vi "Controller_TCrane_MoreData.vi"() -> ()   [LabVIEW 2009]
uses:
  <vilib>/Platform/TimedLoop/XDataNode/nitl_modes.ctl
  Instance           2 23Saved   OpenLoop_TCrane .vi
  <vilib>/Platform/TimedLoop/XDataNode/XDataNode.xnode
  <vilib>/Platform/TimedLoop/XDataNode/loadlvalarms.vi
  <vilib>/Platform/TimedLoop/XDataNode/timing_clust.ctl
  <vilib>/Platform/TimedLoop/XDataNode/wakeup.ctl
  Instance           3 23Saved   OpenLoop_TCrane .vi
  Instance           4 23Saved   OpenLoop_TCrane .vi
  Instance           5 23Saved   OpenLoop_TCrane .vi
  <vilib>/Utility/file.llb/Write To Spreadsheet File (DBL).vi
  <vilib>/Utility/file.llb/Write To Spreadsheet File (string).vi
  Dependences/RTdac/RTDACUSB_TCrane.dll
  <vilib>/Platform/TimedLoop/XDataNode/XDNodeRunTimeDep.lvlib
panel:
  in  "Start saving":bool
  in  "Tab Control":T1(tab)
  out "Controller Description":string
  in  "Motors on":bool caption="Motors"
  out "X displacement chart":dbl(graph)
  out "Y displacement chart":dbl(graph)
  out "Z displacement chart":dbl(graph)
  out "XY Graph":cluster{"Y":dbl[], "Y":dbl[]}[](graph)
  out "Alpha":dbl
  out "Beta":dbl
  in  "Controller:":u8(ring) items=["None", "P (Tracking)", "Self Event Triggered from ED"]
  in  "X":dbl
  in  "Stop Controller":bool
  in  "T":dbl min=0.0 max=3.14 step=0.05
  in  "Z":dbl
  in  "Referense Slide X":dbl(slide) scale=0.0..50.0
  in  "Referense Slide T":dbl(slide) scale=0.0..3.14
  in  "Referense Slide Z":dbl(slide) scale=0.0..100.0
  in  "Cont Switch X":bool
  in  "Cont Switch T":bool
  in  "Cont Switch Z":bool
  in  "stop 2":bool
  in  "Home":bool
  in  "Reset angles":bool
  in  "Motors off":bool
  in  "Saving":bool
  in  "Stop saving":bool
  out "current time":timestamp
  out "Timestamp":dbl format="%#.12g"
  out "Path":path
  out "X Scope":dynamicdata(graph)
  out "Theta Scope":dynamicdata(graph)
  out "Z Scope":dynamicdata(graph)
  out "Waveform Chart":i32(graph)
  out "Counter pulses":dbl format="%#.12g"
  out "Encoder X":dbl format="%#.12g"
  in  "X-axis control":dbl(slide) scale=-1.0..1.0
  in  "X-Motor On/Off":bool
  out "X - Motor On/Off":bool
  out "Numeric":dbl
  out "No of detected boards":dbl
  out "Logic version":dbl
  out "Last error":string
  in  "Theta-angle control":dbl(slide) scale=-1.0..1.0
  in  "T-Motor On/Off":bool
  out "Theta - Motor On/Off":bool
  out "Numeric 2":dbl
  in  "Z-axis control":dbl(slide) scale=-1.0..1.0
  in  "Z-Motor On/Off":bool
  out "Z - Motor On/Off":bool
  out "Numeric 3":dbl
  out "Encoder Theta":dbl format="%#.12g"
  out "Encoder Z":dbl format="%#.12g"
  out "Encoder Alfa":dbl format="%#.12g"
  out "Encoder Beta":dbl format="%#.12g"
  in  "Limit flags":T2(radio)=enum."Radio Selection 2"
  in  "Therm flags":T3(radio)=enum."Radio Selection 2"
  in  "Stop motors":bool
  out "X-axis therm flag":bool
  out "T-angle therm flag":bool
  out "Z-axis therm flag":bool
  out "X-axis limit flag":bool
  out "T-angle limit flag":bool
  out "Z-axis limit flag":bool
  in  "Reset encoders":bool
  out "RESET value":dbl format="%#.12g"
  in  "Soft limit flags":bool=TRUE
  in  "k 1":dbl=0.4 step=0.1
  in  "k 2":dbl=0.4 step=0.1
  in  "Mode":T4=enum."Discard missed periods, maintain original phase"
  out "Sample time [ms]":dbl format="%#.12g"
  out "Self event trigerred Enabled":bool
  out "Event interval":dbl format="%#.12g"
  out "u2":sgl
  out "u1":sgl
  out "Event indicator":bool
  out "Packet Total":u32
  out "Packet Success":u32
  out "TimestampSymb":u32
  out "X Reference":sgl
  out "Y Reference":sgl
  out "X Scope ED":dynamicdata(graph)
  out "Waveform Chart 2":dbl(graph)
  out "Theta Scope ED":dynamicdata(graph)
  out "x1":sgl(graph)
  out "x2":sgl(graph)
  out "x5":sgl(graph)
  out "x6":sgl(graph)
  out "Current Ref Z":dbl
  out "Current Ref X":dbl
  out "Current Ref T":dbl
  in  "Offset Beta":dbl
  in  "Offset Alpha":dbl
  # "RT-DAC/USB status"
  # "Tower Crane motor control"
  # "Controller Parameters"
  # "Default Controllers"
  # "Self Triggered Controller"
  # "Performance Evaluation"
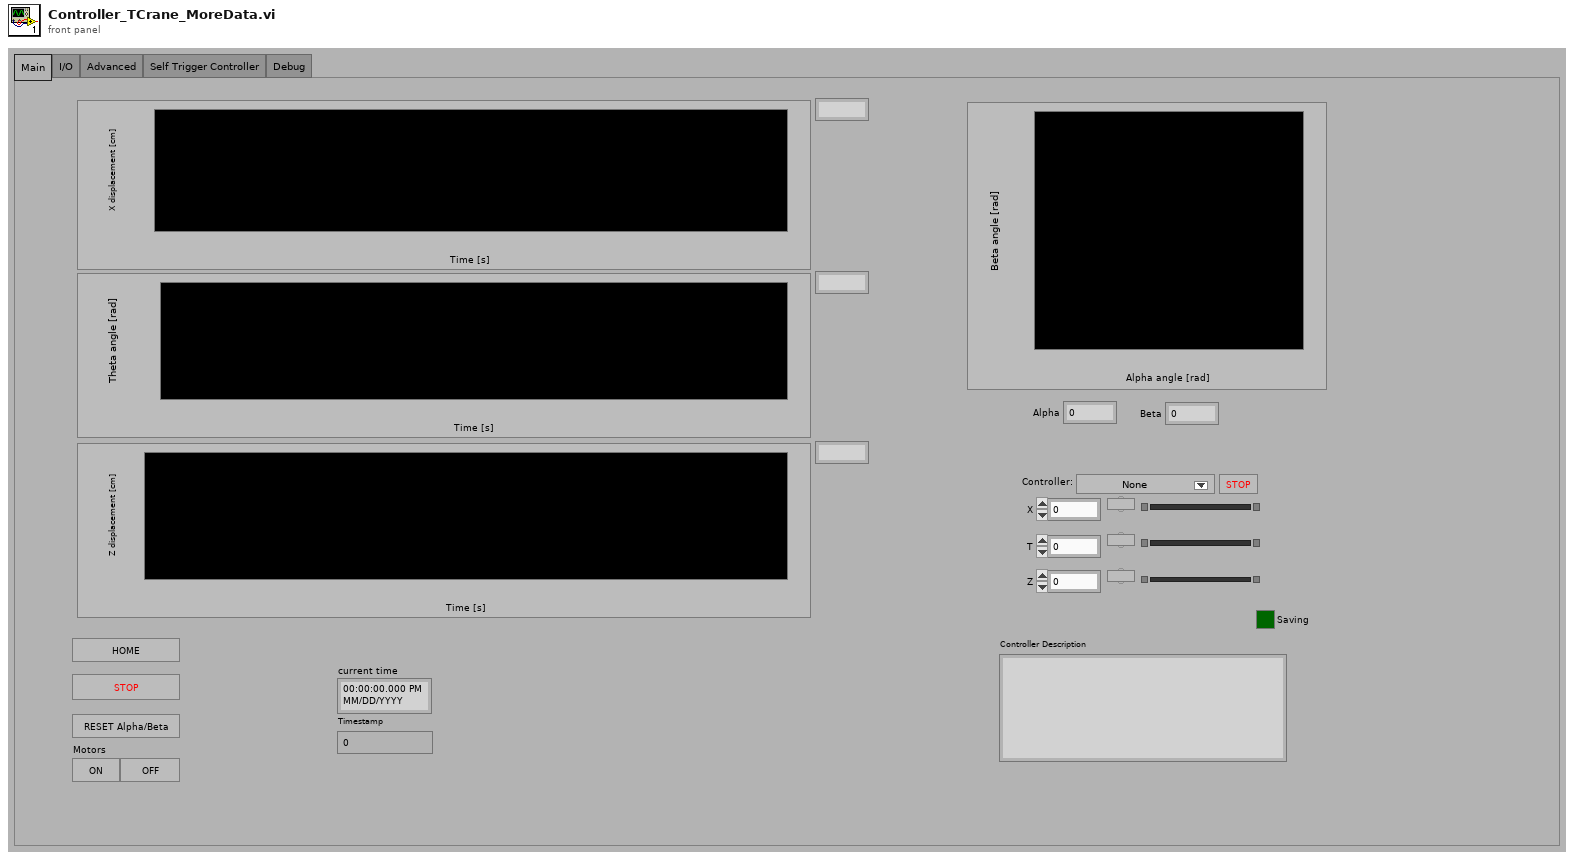
[diagram p1: front panel]
types:
  T1 = enum32{"Main", "I/O", "Advanced", "Self Trigger Controller", "Debug"}
  T2 = enum32{"Set limit flags to:", "Radio Selection 2"}
  T3 = enum32{"Set therm flags to:", "Radio Selection 2"}
  T4 = typedef "XDNodeRunTimeDep.lvlib/nitl_modes.ctl" = enum32{"No Change", "Process missed periods, maintain original phase", "Discard missed periods, maintain original phase", "Process missed periods, ignore original phase", "Discard missed periods, ignore original phase"}
  T5 = typedef "XDNodeRunTimeDep.lvlib/timing_clust.ctl" = cluster{"Expected End [f-1]":u64, "Actual End [f-1]":u64, "Finished Late? [f-1]":bool, "Expected End [i-1]":u64, "Actual End [i-1]":u64, "Finished Late? [i-1]":bool, "Expected Start [i]":u64, "Actual Start [i]":u64, "Expected Start [f]":u64, "Actual Start [f]":u64, "Source Name":string, "Structure Name":string, "Period":i64, "Deadline":i64, "Offset":i64, "Start":i64, "Priority":i32, "Timeout":i32, "Mode":T4, "Wakeup Reason":T6, "Error":errorcluster, "Source Type":string, "Secondary Source Type":string, "Global End Time":u64, "Global Start Time":u64, "Frame Duration":u64, "Iteration Duration":u64, "Assigned CPU":i32, "I/O Scan Engine Mode":u32}
  T6 = typedef "XDNodeRunTimeDep.lvlib/wakeup.ctl" = enum32{"Normal", "Aborted", "Asynchronous wakeup", "Timing source error", "Timed loop error", "Timeout"}
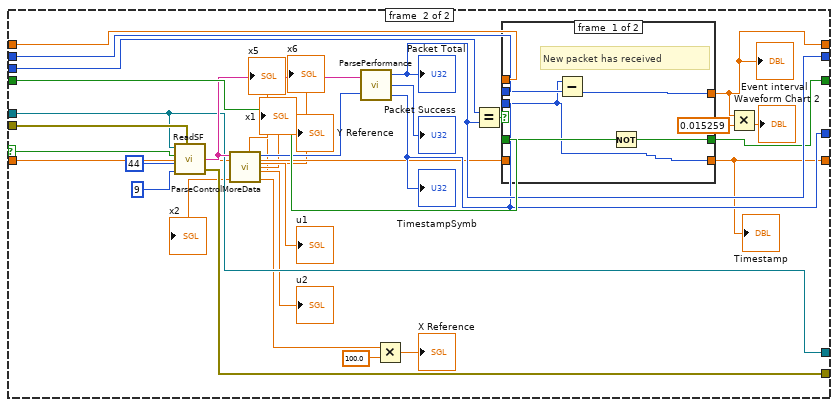
[diagram p2: hidden frame]
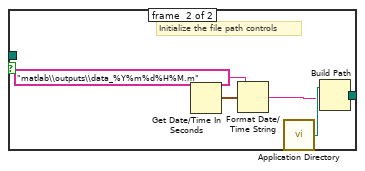
[diagram p4: hidden frame]
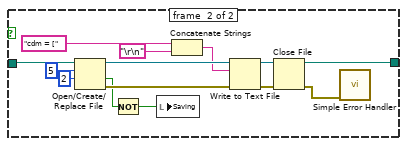
[diagram p5: hidden frame]
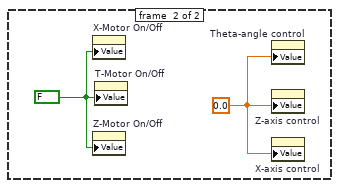
[diagram p6: hidden frame]
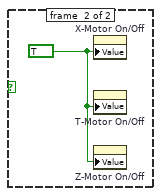
[diagram p7: hidden frame]
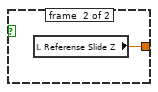
[diagram p8: hidden frame]
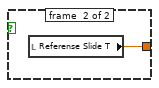
[diagram p9: hidden frame]
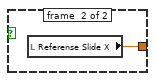
[diagram p10: hidden frame]
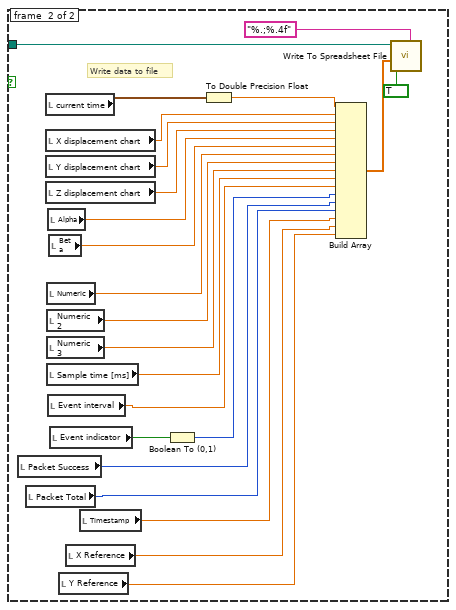
[diagram p11: hidden frame]
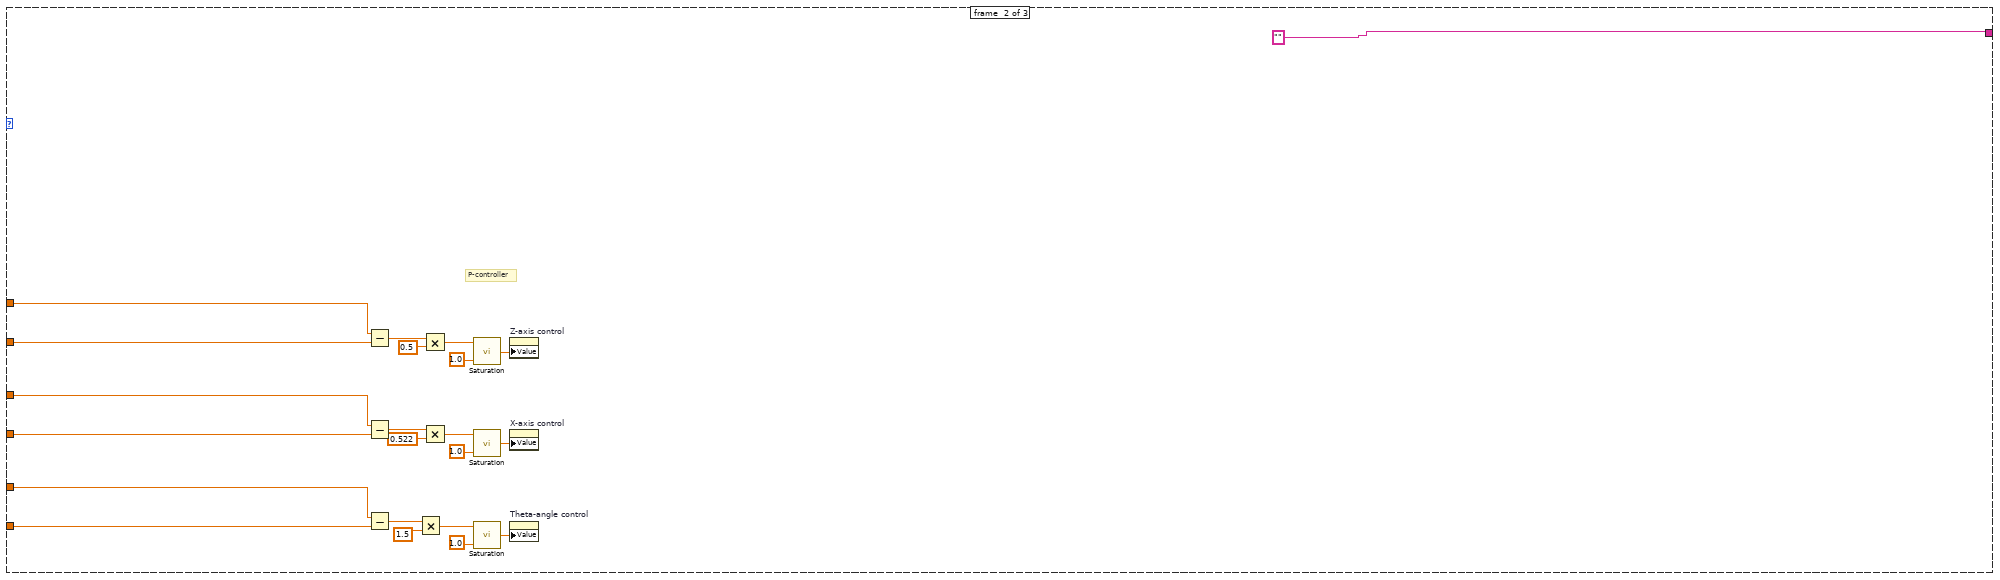
[diagram p12: hidden frame]
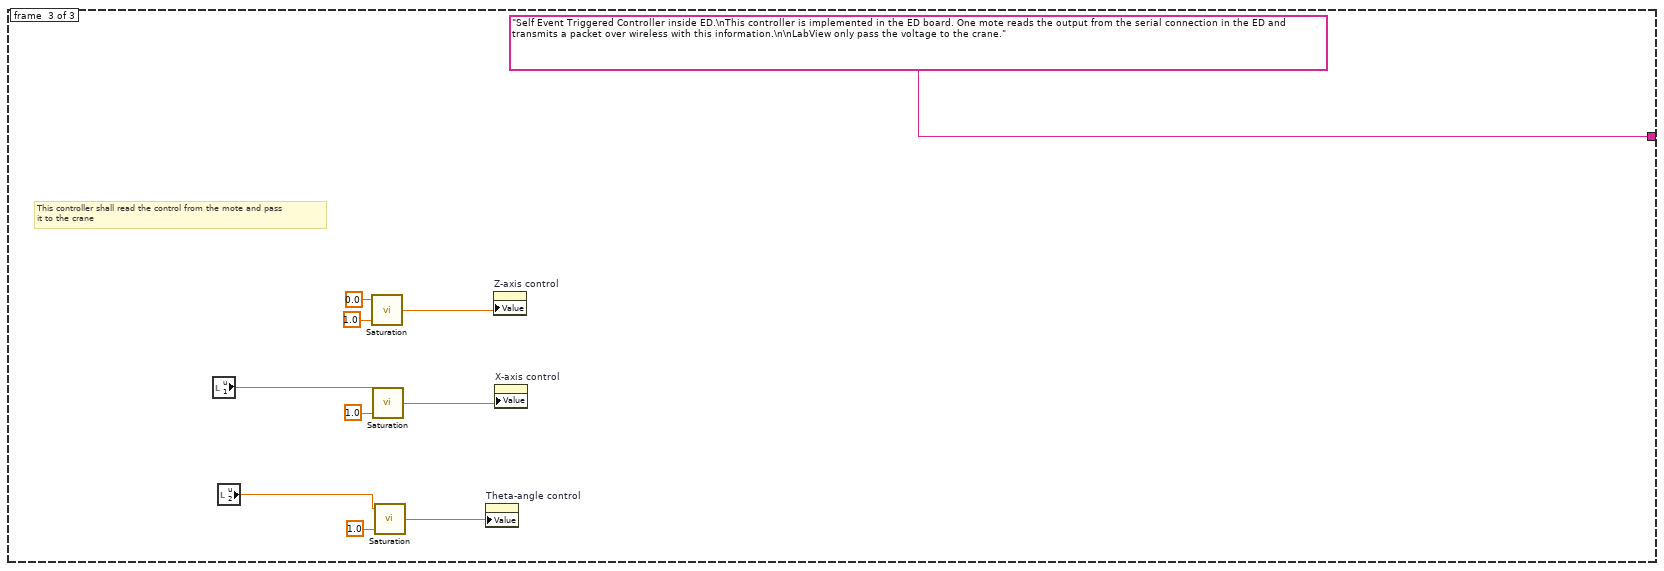
[diagram p13: hidden frame]
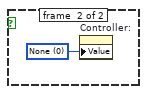
[diagram p14: hidden frame]
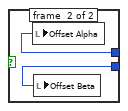
[diagram p15: hidden frame]
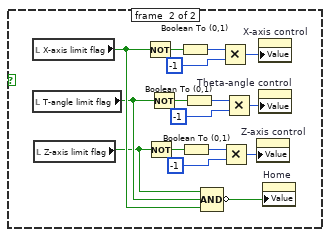
[diagram p16: hidden frame]
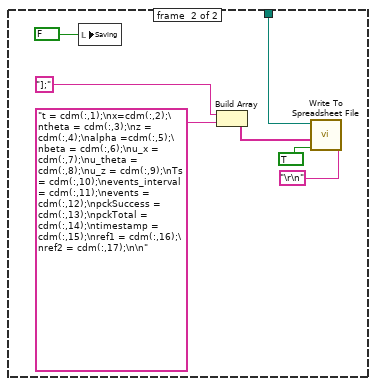
[diagram p17: hidden frame]
diagram:
  (unwired) 0.0
  (unwired) 0.0
  w10 = 0.0
  # "Initialize the file path controls"
  # "Initialize the file path controls"
  n1 = Get Date/Time In Seconds() -> (seconds since 1Jan1904=w9:timestamp)
  n2 = dll-call lib="C:/Documents and Settings/student/Desktop/crane controller/Dependences/RTdac/RTDACUSB_TCrane.dll" fn="RTDACUSB_NoOfDetectedBoards" ("PlxApi.dll:PlxBusIopWrite")() -> ("pNoOfDetectedBoards"=w23:i32)  [unwired: 5 in, 2 out]
  "No of detected boards" <- w23
  n3 = Format Date/Time String(time format string (%c)="matlab\\outputs\\data_%Y%m%d%H%M.m", seconds (now)=w9) -> (date/time string=w6:string)  [unwired: 1 in]
  n4 = call <vilib>:"Application Directory.vi"() -> ("Application Directory"=w17:path)
  n5 = Build Path(base path=w17, name or relative path=w6) -> (appended path=w7:path)
  n6 = Less?(x=w23, y=1) -> (x < y?=w22:bool)
  n7 = local write "Path"(w7) -> ()
  n8 = call "Display Message to User"("Enable"=w22) -> ("OK"=w11:bool)  [unwired: 9 in, 1 out]
  n9 = Get Date/Time In Seconds() -> (seconds since 1Jan1904=w4:timestamp)
  n10 = call "OpenSF.vi"() -> ("error out"=w15:errorcluster, "connection ID"=w16:refnum<k5>)  [unwired: 1 out]
  n11 = Format Date/Time String(time format string (%c)="matlab\\outputs\\data_%Y%m%d%H%M.m", seconds (now)=w4) -> (date/time string=w2:string)  [unwired: 1 in]
  n12 = call <vilib>:"Application Directory.vi"() -> ("Application Directory"=w5:path)
  n13 = while {
    tunnel: w16 -> [w51]
    tunnel: w15 -> [w50]
    tunnel: [w49] -> w14
    tunnel: [w48] -> w13
    shift-right: [w40] -> _
    shift-left: FALSE -> [w45]
    shift-right: [w44] -> _
    shift-left: _ -> [w43]
    shift-right: [w42] -> _
    shift-left: _ -> [w41]
    shift-right: [w38] -> _
    shift-left: w10 -> [w39]
    shift-right: [w25] -> _
    shift-left: w10 -> [w24]
    stop <- TRUE continue-if-true
    # "Feed control signals, reference signals and measurements into the scopes"
    # "Read data from the Serial Forwarer (motes)"
    n14 = local read "Self event trigerred Enabled"() -> (w47:bool)
    n15 = case shown="True" w47 {
      selector: w47 -> [_ w65]
      tunnel: w51 -> [w57 w83]
      tunnel: w50 -> [w56 w88]
      tunnel: [w57 w83] -> w49
      tunnel: [w56 w89] -> w48
      tunnel: w45 -> [w55 w86]
      tunnel: [w55 w76] -> w40
      tunnel: [w54 w74] -> w44
      tunnel: w43 -> [w54 w73]
      tunnel: [_ w79] -> w42
      tunnel: w41 -> [_ w78]
      tunnel: [w53 w59] -> w38
      tunnel: w39 -> [w53 w75]
      tunnel: [w52 w67] -> w25
      tunnel: w24 -> [w52 w66]
      frame #0 {
      }
      frame #1 {
        n16 = call "ReadSF.vi"("connection ID in"=w83, "enabled"=w65, "bytes to read"=44 ("f"), "header size"=9 ("bytes to read"), "error in"=w88) -> ("string"=w85:string, "error out"=w89:errorcluster)  [unwired: 1 out]
        n17 = call "ParseControlMoreData.vi"("data out"=w85) -> ("ref1"=w69:sgl, "u2"=→"u2":sgl, "u1"=→"u1":sgl, "Bytes read"=w72:i32, "ref2"=→"Y Reference":sgl, "x1"=→"x1":sgl, "x2"=→"x2":sgl, "x5"=→"x5":sgl, "x6"=→"x6":sgl)
        n18 = call "ParsePerformance.vi"("data out"=w85, "offset"=w72) -> ("pckTotal"=w79:u32, "pckSuccess"=→"Packet Success":u32, "timestamp"=w74:u32)
        "Packet Total" <- w79
        "TimestampSymb" <- w74
        n19 = Multiply(x=w69, y=sgl 100.0) -> (x*y=→"X Reference":sgl)
        n20 = Equal?(x=w78, y=w79) -> (x = y?=w77:bool)
        n21 = case shown="True" w77 {
          tunnel: w86 -> [w94 w97]
          tunnel: [w93 w97] -> w76
          tunnel: w75 -> [_ w96]
          tunnel: [w91 w96] -> w59
          tunnel: w74 -> [w90 _]
          tunnel: w73 -> [w92 _]
          tunnel: [w90 w95] -> w67
          tunnel: w66 -> [_ w95]
          frame #0 {
            # "New packet has received"
            n22 = Subtract(x=w90, y=w92) -> (x-y=w91:u32)
            n23 = Not(x=w94) -> (.not. x?=w93:bool)
          }
          frame #1 {
          }
        }
        "Event interval" <- w59
        "Timestamp" <- w67
        n24 = Multiply(x=w59, y=0.015259) -> (x*y=→"Waveform Chart 2":dbl)
      }
    }
    "Event indicator" <- w40
    n25 = local read "X Reference"() -> (w33:sgl)
    n26 = local read "Y Reference"() -> (w27:sgl)
    n27 = local read "Y displacement chart"() -> (w30:dbl)
    n28 = local read "X displacement chart"() -> (w26:dbl)
    n29 = local read "u2"() -> (w28:sgl)
    n30 = local read "u1"() -> (w36:sgl)
    n31 = Multiply(x=w28, y=5) -> (x*y=w31:sgl)
    n32 = Multiply(x=w36, y=40) -> (x*y=w34:sgl)
    n33 = Merge Signals(w30, w27, w31) -> (→"Theta Scope ED":dynamicdata)
    n34 = Merge Signals(w26, w33, w34) -> (→"X Scope ED":dynamicdata)
  }
  n35 = Build Path(base path=w5, name or relative path=w2) -> (appended path=w1:path)
  n36 = node-c288("Mode") -> (w20:T5)  [unwired: 9 in]
  n37 = timed-loop {
    tunnel: w11 -> [w289]
    timing: w20 -> [_]
    timing-out: [_] -> w19
    shift-right: [w101] -> _
    shift-left: w1 -> [w99]
    stop <- w290 stop-if-true
    w135 = 0.00153
    w238 = 0.00153
    w276 = 1
    w136 = 0
    # "It enabled to read from the mote"
    # "Plot the values from the Wireless sensor"
    # "Stop saving of data"
    # "Turn off all the motors"
    # "Turn on all the motors"
    # "Get reference signals"
    # "Take crane to home position"
    # "Stop the controller"
    # "Feed control signals, reference signals and measurements into the scopes"
    n38 = node-c288() -> ()  [unwired: 1 in, 1 out]
    n39 = Get Date/Time In Seconds() -> (seconds since 1Jan1904=w120:timestamp)
    "current time" <- w120
    n40 = local read "Stop Controller"() -> (w141:bool)
    n41 = local read "Stop motors"() -> (w140:bool)
    n42 = Compound Arithmetic op=OR(w141, "Motors off", w140) -> (w143:bool)
    n43 = dll-call lib="C:/Documents and Settings/student/Desktop/crane controller/Dependences/RTdac/RTDACUSB_TCrane.dll" fn="RTDACUSB_Receive" ("PlxApi.dll:PlxBusIopWrite")("pLogicVersion"=w136, "pApplicationName"="TestInTeCo", "pCN1Direction"=w136, "pCN1Input"=w136, "pPWMDivider"=w136, "pPWMWidth0"=w136, "pPWMWidth1"=w136, "pPWMWidth2"=w136, "pPWMDir0"=w136, "pPWMDir1"=w136, "pPWMDir2"=w136, "pPWMBrake0"=w136, "pPWMBrake1"=w136, "pPWMBrake2"=w136, "pPWMTherm0"=w136, "pPWMTherm1"=w136, "pPWMTherm2"=w136, "pPWMThermFlag0"=w136, "pPWMThermFlag1"=w136, "pPWMThermFlag2"=w136, "pNOFlag"=w136, "pLimitActive0"=w136, "pLimitActive1"=w136, "pLimitActive2"=w136, "pLimitFlag0"=w136, "pLimitFlag1"=w136, "pLimitFlag2"=w136, "pLimit0"=w136, "pLimit1"=w136, "pLimit2"=w136, "pEncoderReset0"=w136, "pEncoderReset1"=w136, "pEncoderReset2"=w136, "pEncoderReset3"=w136, "pEncoderReset4"=w136, "pEncoderAutoResetFlag0"=w136, "pEncoderAutoResetFlag1"=w136, "pEncoderAutoResetFlag2"=w136, "pEncoder0"=w136, "pEncoder1"=w136, "pEncoder2"=w136, "pEncoder3"=w136, "pEncoder4"=w136, "pTmrCnt0_Reset"=w136, "pTmrCnt0_Mode"=w136, "pTmrCnt0_Counter"=w136) -> ("pLogicVersion"=→"Logic version":u32, "pPWMThermFlag0"=w257:u32, "pPWMThermFlag1"=w258:u32, "pPWMThermFlag2"=w259:u32, "pLimitActive0"=w237:u32, "pLimitActive1"=w235:u32, "pLimitActive2"=w236:u32, "pEncoder0"=w129:i32, "pEncoder1"=w127:i32, "pEncoder2"=w125:i32, "pEncoder3"=w204:i32, "pEncoder4"=w203:i32, "pTmrCnt0_Counter"=w281:u32)  [unwired: 37 in, 2 out]
    "Counter pulses" <- w281
    "Encoder X" <- w129
    "Encoder Theta" <- w127
    "Encoder Z" <- w125
    n44 = case shown="True" "Reset angles" {
      tunnel: w204 -> [_ w389]
      tunnel: w203 -> [_ w388]
      frame #0 {
      }
      frame #1 {
        n45 = local write "Offset Alpha"(w389) -> ()
        n46 = local write "Offset Beta"(w388) -> ()
      }
    }
    n47 = case shown="True" w143 {
      frame #0 {
      }
      frame #1 {
        w318 = 0.0 ("Theta-angle control")
        w319 = FALSE ("T-Motor On/Off")
        n48 = property on="X-Motor On/Off" class="Bool (strict)"("Value"=w319) -> ()  [unwired: 2 in, 2 out]
        n49 = property on="Z-Motor On/Off" class="Bool (strict)"("Value"=w319) -> ()  [unwired: 2 in, 2 out]
        n50 = property on="T-Motor On/Off" class="Bool (strict)"("Value"=w319) -> ()  [unwired: 2 in, 2 out]
        n51 = property on="Theta-angle control" class="Slide (strict)"("Value"=w318) -> ()  [unwired: 2 in, 2 out]
        n52 = property on="Z-axis control" class="Slide (strict)"("Value"=w318) -> ()  [unwired: 2 in, 2 out]
        n53 = property on="X-axis control" class="Slide (strict)"("Value"=w318) -> ()  [unwired: 2 in, 2 out]
      }
    }
    n54 = case shown="True" "Motors on" {
      frame #0 {
      }
      frame #1 {
        w320 = TRUE ("X-Motor On/Off")
        n55 = property on="X-Motor On/Off" class="Bool (strict)"("Value"=w320) -> ()  [unwired: 2 in, 2 out]
        n56 = property on="T-Motor On/Off" class="Bool (strict)"("Value"=w320) -> ()  [unwired: 2 in, 2 out]
        n57 = property on="Z-Motor On/Off" class="Bool (strict)"("Value"=w320) -> ()  [unwired: 2 in, 2 out]
      }
    }
    n58 = case shown="True" "Stop Controller" {
      frame #0 {
      }
      frame #1 {
        w387 = u16 0 items=["None", "P"] ("Controller:")
        n59 = property on="Controller:" class="Ring (strict)"("Value"=w387) -> ()  [unwired: 2 in, 2 out]
      }
    }
    n60 = Greater?(x=w257, y=1) -> (0:→"X-axis therm flag":bool)
    n61 = Less?(x=w237, y=1) -> (x < y?=→"X-axis limit flag":bool)
    n62 = Less?(x=w235, y=1) -> (x < y?=→"T-angle limit flag":bool)
    n63 = Less?(x=w236, y=1) -> (x < y?=→"Z-axis limit flag":bool)
    n64 = Greater?(x=w258, y=1) -> (0:→"T-angle therm flag":bool)
    n65 = Greater?(x=w259, y=1) -> (0:→"Z-axis therm flag":bool)
    n66 = Multiply(x=w125, y=0.00995) -> (x*y=→"Z displacement chart":dbl)
    n67 = Multiply(x=w127, y=0.00157) -> (x*y=→"Y displacement chart":dbl)
    n68 = Subtract(x=w204, y="Offset Alpha") -> (x-y=w132:dbl)
    "Encoder Alfa" <- w132
    n69 = Subtract(x=w203, y="Offset Beta") -> (x-y=w134:dbl)
    "Encoder Beta" <- w134
    n70 = Multiply(x=w129, y=0.00582) -> (x*y=→"X displacement chart":dbl)
    n71 = local read "Encoder Beta"() -> (w239:dbl)
    n72 = local read "Encoder Alfa"() -> (w240:dbl)
    n73 = Multiply(x=w240, y=w238) -> (x*y=w242:dbl)
    n74 = Multiply(x=w239, y=w238) -> (x*y=w241:dbl)
    n75 = To Double Precision Float(number=w281) -> (double precision float=w288:dbl)
    n76 = To Double Precision Float(number=w120) -> (double precision float=w123:dbl)
    n77 = Multiply(x=w134, y=w135) -> (x*y=→"Beta":dbl)
    n78 = while {
      shift-right: [w317] -> w122
      shift-left: _ -> [w316]
      tunnel: w123 -> [w317]
      tunnel: [w316] -> w121
      tunnel: FALSE -> [w315]
      stop <- w315 continue-if-true
    }
    n79 = Multiply(x=w132, y=w135) -> (x*y=→"Alpha":dbl)
    n80 = for {
      N: 10 -> [_]
      tunnel: w241 -> [w413]
      tunnel: w242 -> [w414]
      tunnel: [w414] -> w249 mode=indexing
      tunnel: [w413] -> w248 mode=indexing
    }
    n81 = while {
      shift-right: [w417] -> w287
      shift-left: _ -> [w416]
      tunnel: w288 -> [w417]
      tunnel: [w416] -> w286
      tunnel: FALSE -> [w415]
      stop <- w415 continue-if-true
    }
    n82 = Subtract(x=w122, y=w121) -> (x-y=w118:dbl)
    n83 = call "Convert to Dynamic Data"("Array"=w249) -> ("Dynamic Data Type"=w250:dynamicdata)  [unwired: 3 in]
    n84 = call "Convert to Dynamic Data2"("Array"=w248) -> ("Dynamic Data Type"=w252:dynamicdata)  [unwired: 3 in]
    n85 = Multiply(x=w118, y=1000.0) -> (x*y=w116:dbl)
    "Sample time [ms]" <- w116
    n86 = Subtract(x=w287, y=w286) -> (x-y=w285:dbl)
    n87 = call "Build XY Graph"("Y Input"=w252, "X Input"=w250) -> ("XY Graph"=→"XY Graph":cluster{"Y":dbl[], "Y":dbl[]}[])  [unwired: 8 in, 1 out]
    n88 = Divide(x=w285, y=40000) -> ()  [unwired: 1 out]
    n89 = Or(x=w289, y="stop 2") -> (x .or. y?=w290:bool)
    n90 = To Long Integer(number=w116) -> (32bit integer=→"Waveform Chart":i32)
    n91 = Stop(stop? (T)=w290) -> ()
    n92 = Or(x="Stop saving", y=w290) -> (x .or. y?=w213:bool)
    n93 = And(x="Saving", y=w213) -> (x .and. y?=w124:bool)
    n94 = local read "Saving"() -> (w114:bool)
    n95 = Not(x=w114) -> (.not. x?=w115:bool)
    n96 = And(x="Start saving", y=w115) -> (x .and. y?=w98:bool)
    n97 = case shown="True" w98 {
      tunnel: [w291 w292] -> w100
      tunnel: w99 -> [w291 _]
      frame #0 {
      }
      frame #1 {
        # "Initialize the file path controls"
        n98 = Get Date/Time In Seconds() -> (seconds since 1Jan1904=w295:timestamp)
        n99 = Format Date/Time String(time format string (%c)="matlab\\outputs\\data_%Y%m%d%H%M.m", seconds (now)=w295) -> (date/time string=w293:string)  [unwired: 1 in]
        n100 = call <vilib>:"Application Directory.vi"() -> ("Application Directory"=w296:path)
        n101 = Build Path(base path=w296, name or relative path=w293) -> (appended path=w292:path)
      }
    }
    "Path" <- w100
    n102 = flat-sequence {
      tunnel: [w299] -> w101
      tunnel: w98 -> [w298]
      tunnel: w100 -> [w297]
      frame #0 {
        # "Initialize saving of data"
        n103 = case shown="True" w298 {
          tunnel: w297 -> [w300 w306]
          tunnel: [w300 w303] -> w299
          frame #0 {
          }
          frame #1 {
            n104 = Open/Create/Replace File(file path (use dialog)=w306, operation (0:open)=5, access (0:read/write)=2) -> (refnum out=w312:refnum<file>, cancelled=w305:bool, error out=w309:errorcluster)  [unwired: 3 in]
            n105 = Not(x=w305) -> (.not. x?=w301:bool)
            n106 = local write "Saving"(w301) -> ()
            n107 = Concatenate Strings("cdm = [", "\r\n") -> (w308:string)
            n108 = Write to Text File(file (use dialog)=w312, text=w308, error in=w309) -> (refnum out=w311:refnum<file>, error out=w310:errorcluster)  [unwired: 1 in, 1 out]
            n109 = Close File(refnum=w311, error in=w310) -> (path=w303:path, error out=w302:errorcluster)
            n110 = call <vilib>:"Simple Error Handler.vi"("error in (no error)"=w302) -> ()  [unwired: 4 in, 5 out]
          }
        }
      }
    }
    n111 = local read "Stop Controller"() -> (w196:bool)
    n112 = local read "Stop motors"() -> (w198:bool)
    n113 = local read "T-angle limit flag"() -> (w230:bool)
    n114 = case shown="True" w124 {
      tunnel: w101 -> [_ w410]
      frame #0 {
      }
      frame #1 {
        n115 = local write "Saving"(FALSE) -> ()
        n116 = Build Array("];", "t = cdm(:,1);\nx=cdm(:,2);\ntheta = cdm(:,3);\nz = cdm(:,4);\nalpha =cdm(:,5);\nbeta = cdm(:,6);\nu_x = cdm(:,7);\nu_theta = cdm(:,8);\nu_z = cdm(:,9);\nTs = cdm(:,10);\nevents_interval = cdm(:,11);\nevents = cdm(:,12);\npckSuccess = cdm(:,13);\npckTotal = cdm(:,14);\ntimestamp = cdm(:,15);\nref1 = cdm(:,16);\nref2 = cdm(:,17);\n\n") -> (w409:string[])
        n117 = call-poly <vilib>:"Write To Spreadsheet File.vi"("delimiter (\\t)"="\r\n", "append to file? (new file:F)"=TRUE, "1D data"=w409, "file path (dialog if empty)"=w410) -> ()  [unwired: 4 in, 1 out]
      }
    }
    n118 = local read "Limit flags"() -> (w233:T2)
    n119 = local read "Soft limit flags"() -> (w209:bool)
    n120 = Or(x=w196, y=w198) -> (x .or. y?=w197:bool)
    n121 = feedback #1() -> (w155:dbl)  [unwired: 1 in]
    n122 = call "LimitFlagActionSoftLinearizedT.vi"("Soft"=w209, "Axis limit flag"=w230, "Old Control"=w155, "Global limit flag active"=w233, "Stop motors global"=w197, "Stop motor local"="T-Motor On/Off", "Axis control signal"="Theta-angle control") -> ("Slider control"=w154:dbl, "PWM Brake"=w229:u32, "PWM Direction"=w228:u32, "PWM width"=w227:u32)
    n123 = local read "Stop Controller"() -> (w193:bool)
    n124 = local read "X-axis limit flag"() -> (w220:bool)
    n125 = local read "Stop motors"() -> (w195:bool)
    n126 = local read "Soft limit flags"() -> (w208:bool)
    n127 = local read "Limit flags"() -> (w221:T2)
    n128 = local read "Stop Controller"() -> (w199:bool)
    n129 = Or(x=w193, y=w195) -> (x .or. y?=w194:bool)
    n130 = local read "Z-axis limit flag"() -> (w158:bool)
    n131 = local read "Limit flags"() -> (w224:T2)
    n132 = feedback #2() -> (w153:dbl)  [unwired: 1 in]
    n133 = call "LimitFlagActionSoftLinearizedX.vi"("Soft"=w208, "Axis limit flag"=w220, "Old Control"=w153, "Global limit flag active"=w221, "Stop motors global"=w194, "Stop motor local"="X-Motor On/Off", "Axis control signal"="X-axis control") -> ("Slider control"=w152:dbl, "PWM Brake"=w217:u32, "PWM Direction"=w216:u32, "PWM width"=w215:u32)
    n134 = local read "Cont Switch T"() -> (w162:bool)
    n135 = local read "Cont Switch X"() -> (w164:bool)
    n136 = local read "Cont Switch Z"() -> (w160:bool)
    n137 = Or(x=w199, y="Stop motors") -> (x .or. y?=w200:bool)
    n138 = case shown="False" w162 {
      tunnel: [w325 w326] -> w161
      frame #0 {
        n139 = local read "T"() -> (w325:dbl)
      }
      frame #1 {
        n140 = local read "Referense Slide T"() -> (w326:dbl)
      }
    }
    n141 = case shown="False" w164 {
      tunnel: [w327 w328] -> w163
      frame #0 {
        n142 = local read "X"() -> (w327:dbl)
      }
      frame #1 {
        n143 = local read "Referense Slide X"() -> (w328:dbl)
      }
    }
    n144 = case shown="False" w160 {
      tunnel: [w323 w324] -> w159
      frame #0 {
        n145 = local read "Z"() -> (w323:dbl)
      }
      frame #1 {
        n146 = local read "Referense Slide Z"() -> (w324:dbl)
      }
    }
    n147 = feedback #3() -> (w157:dbl)  [unwired: 1 in]
    n148 = call "LimitFlagActionSoftLinearizedZ.vi"("Soft"="Soft limit flags", "Axis limit flag"=w158, "Old Control"=w157, "Global limit flag active"=w224, "Stop motors global"=w200, "Stop motor local"="Z-Motor On/Off", "Axis control signal"="Z-axis control") -> ("Slider control"=w156:dbl, "PWM Brake"=w151:u32, "PWM Direction"=w226:u32, "PWM width"=w225:u32)
    n149 = dll-call lib="C:/Documents and Settings/student/Desktop/crane controller/Dependences/RTdac/RTDACUSB_TCrane.dll" fn="RTDACUSB_LastError" ("PlxApi.dll:PlxBusIopWrite")() -> ("dsrp"=→"Last error":string)  [unwired: 3 in, 2 out]
    n150 = Boolean To (0,1)(Boolean="Reset encoders") -> (0, 1=w246:i16)
    "RESET value" <- w246
    n151 = local read "X displacement chart"() -> (w179:dbl)
    n152 = local read "X-axis control"() -> (w173:dbl)
    n153 = local read "Y displacement chart"() -> (w177:dbl)
    n154 = local read "Z displacement chart"() -> (w175:dbl)
    n155 = local read "Theta-angle control"() -> (w170:dbl)
    n156 = local read "Z-axis control"() -> (w167:dbl)
    n157 = dll-call lib="C:/Documents and Settings/student/Desktop/crane controller/Dependences/RTdac/RTDACUSB_TCrane.dll" fn="RTDACUSB_Send" ("PlxApi.dll:PlxBusIopWrite")("PWMDivider"=10, "PWMWidth0"=w215, "PWMWidth1"=w227, "PWMWidth2"=w225, "PWMDir0"=w216, "PWMDir1"=w228, "PWMDir2"=w226, "PWMBrake0"=w217, "PWMBrake1"=w229, "PWMBrake2"=w151, "PWMThermFlag0"="Therm flags", "PWMThermFlag1"="Therm flags", "PWMThermFlag2"="Therm flags", "LimitFlag0"="Limit flags", "LimitFlag1"="Limit flags", "LimitFlag2"="Limit flags", "Limit0"=133, "Limit1"=29, "Limit2"=156, "EncoderReset0"=w246, "EncoderReset1"=w246, "EncoderReset2"=w246, "EncoderReset3"=w246, "EncoderReset4"=w246, "EncoderAutoResetFlag0"=w276, "EncoderAutoResetFlag1"=w276, "EncoderAutoResetFlag2"=w276, "TmrCnt0_Reset"=0, "TmrCnt0_Mode"=1) -> ()  [unwired: 33 in, 2 out]
    n158 = Multiply(x=w173, y=40) -> (x*y=w171:dbl)
    n159 = Multiply(x=w170, y=5) -> (x*y=w168:dbl)
    n160 = Multiply(x=w167, y=20) -> (x*y=w165:dbl)
    n161 = Merge Signals(w177, w161, w168) -> (→"Theta Scope":dynamicdata)
    n162 = Merge Signals(w175, w159, w165) -> (→"Z Scope":dynamicdata)
    n163 = Merge Signals(w179, w163, w171) -> (→"X Scope":dynamicdata)
    n164 = stacked-sequence {
      tunnel: w101 -> [w329]
      frame #0 {
        n165 = local read "Saving"() -> (w330:bool)
        n166 = case shown="True" w330 {
          tunnel: w329 -> [_ w352]
          frame #0 {
          }
          frame #1 {
            # "Write data to file"
            n167 = local read "Packet Success"() -> (w337:u32)
            n168 = local read "Packet Total"() -> (w336:u32)
            n169 = local read "current time"() -> (w332:timestamp)
            n170 = local read "X displacement chart"() -> (w350:dbl)
            n171 = local read "Y displacement chart"() -> (w349:dbl)
            n172 = local read "Z displacement chart"() -> (w348:dbl)
            n173 = local read "Numeric"() -> (w346:dbl)
            n174 = local read "Numeric 2"() -> (w345:dbl)
            n175 = local read "Numeric 3"() -> (w344:dbl)
            n176 = local read "Sample time [ms]"() -> (w343:dbl)
            n177 = local read "Alpha"() -> (w342:dbl)
            n178 = local read "Event interval"() -> (w339:dbl)
            n179 = local read "Beta"() -> (w341:dbl)
            n180 = local read "Event indicator"() -> (w340:bool)
            n181 = local read "Y Reference"() -> (w333:sgl)
            n182 = local read "X Reference"() -> (w334:sgl)
            n183 = local read "Timestamp"() -> (w335:dbl)
            n184 = Boolean To (0,1)(Boolean=w340) -> (0, 1=w338:i16)
            n185 = To Double Precision Float(number=w332) -> (double precision float=w331:dbl)
            n186 = Build Array(w331, w350, w349, w348, w342, w341, w346, w345, w344, w343, w339, w338, w337, w336, w335, w334, w333) -> (w351:dbl[])
            n187 = call-poly <vilib>:"Write To Spreadsheet File.vi"("format (%.3f)"="%.;%.4f", "append to file? (new file:F)"=TRUE, "1D data"=w351, "file path (dialog if empty)"=w352) -> ()  [unwired: 4 in, 1 out]
          }
        }
      }
    }
    n188 = local read "Start saving"() -> (w107:bool)
    n189 = local read "Saving"() -> (w102:bool)
    n190 = Not(x=w102) -> (.not. x?=w103:bool)
    n191 = local read "Y displacement chart"() -> (w190:dbl)
    n192 = Greater Or Equal?(x="Controller:", y=u8 2) -> (x >= y?=w104:bool)
    "Self event trigerred Enabled" <- w104
    n193 = Exclusive Or(1:w107, 2:w104) -> (0:w108:bool)
    n194 = And(x=w108, y=w103) -> (x .and. y?=w106:bool)
    n195 = local write "Start saving"(w106) -> ()
    n196 = local read "Z displacement chart"() -> (w192:dbl)
    n197 = local read "X displacement chart"() -> (w191:dbl)
    n198 = Not(x=w104) -> (.not. x?=w105:bool)
    n199 = local read "Stop saving"() -> (w111:bool)
    n200 = Select(t="Referense Slide X", s="Cont Switch X", f="X") -> (s? t:f=w150:dbl)
    "Current Ref X" <- w150
    n201 = Select(t="Referense Slide T", s="Cont Switch T", f="T") -> (s? t:f=w186:dbl)
    "Current Ref T" <- w186
    n202 = Select(t="Referense Slide Z", s="Cont Switch Z", f="Z") -> (s? t:f=w149:dbl)
    "Current Ref Z" <- w149
    n203 = local read "Saving"() -> (w110:bool)
    n204 = Exclusive Or(1:w111, 2:w105) -> (0:w112:bool)
    n205 = And(x=w112, y=w110) -> (x .and. y?=w109:bool)
    n206 = local write "Stop saving"(w109) -> ()
    n207 = case shown="True" "Home" {
      frame #0 {
      }
      frame #1 {
        n208 = local read "X-axis limit flag"() -> (w393:bool)
        n209 = local read "T-angle limit flag"() -> (w392:bool)
        n210 = local read "Z-axis limit flag"() -> (w391:bool)
        n211 = Not(x=w393) -> (.not. x?=w403:bool)
        n212 = Not(x=w391) -> (.not. x?=w396:bool)
        n213 = Not(x=w392) -> (.not. x?=w400:bool)
        n214 = Boolean To (0,1)(Boolean=w403) -> (0, 1=w405:i16)
        n215 = Boolean To (0,1)(Boolean=w396) -> (0, 1=w397:i16)
        n216 = Boolean To (0,1)(Boolean=w400) -> (0, 1=w401:i16)
        n217 = Compound Arithmetic op=AND(w391, w392, w393) -> (invert w390:bool)
        n218 = Multiply(x=w405, y=-1) -> (x*y=w404:i32)
        n219 = Multiply(x=w397, y=-1) -> (x*y=w394:i32)
        n220 = Multiply(x=w401, y=-1) -> (x*y=w398:i32)
        n221 = property on="Z-axis control" class="Slide (strict)"("Value"=w394) -> ()  [unwired: 2 in, 2 out]
        n222 = property on="X-axis control" class="Slide (strict)"("Value"=w404) -> ()  [unwired: 2 in, 2 out]
        n223 = property on="Theta-angle control" class="Slide (strict)"("Value"=w398) -> ()  [unwired: 2 in, 2 out]
        n224 = property on="Home" class="Bool (strict)"("Value"=w390) -> ()  [unwired: 2 in, 2 out]
      }
    }
    n225 = local read "Alpha"() -> (w146:dbl)
    n226 = local read "Beta"() -> (w145:dbl)
    n227 = case shown="1" "Controller:" {
      tunnel: w191 -> [_ w375 _]
      tunnel: w150 -> [_ w376 _]
      tunnel: w186 -> [_ w365 _]
      tunnel: w190 -> [_ w364 _]
      tunnel: w149 -> [_ w358 _]
      tunnel: w192 -> [_ w357 _]
      tunnel: "k 1" -> [_ _ _]
      tunnel: "k 2" -> [_ _ _]
      tunnel: w146 -> [_ _ _]
      tunnel: w145 -> [_ _ _]
      tunnel: ["" "" "Self Event Triggered Controller inside ED.\nThis controller is implemented in the ED board. One mote reads the output from the serial connection in the ED and transmits a packet over wireless with this information.\n\nLabView only pass the voltage to the crane."] -> w137
      frame #0 {
        # "No controller"
      }
      frame #1 {
        # "P-controller"
        n228 = Subtract(x=w358, y=w357) -> (x-y=w362:dbl)
        n229 = Subtract(x=w376, y=w375) -> (x-y=w374:dbl)
        n230 = Subtract(x=w365, y=w364) -> (x-y=w369:dbl)
        n231 = Multiply(x=w369, y=1.5) -> (x*y=w367:dbl)
        n232 = Multiply(x=w362, y=0.5) -> (x*y=w360:dbl)
        n233 = Multiply(x=w374, y=0.522) -> (x*y=w371:dbl)
        n234 = call "Saturation.vi"("Limit"=1.0, "Input"=w360) -> ("Output"=w356:dbl)
        n235 = call "Saturation.vi"("Limit"=1.0, "Input"=w371) -> ("Output"=w372:dbl)
        n236 = call "Saturation.vi"("Limit"=1.0, "Input"=w367) -> ("Output"=w363:dbl)
        n237 = property on="Z-axis control" class="Slide (strict)"("Value"=w356) -> ()  [unwired: 2 in, 2 out]
        n238 = property on="X-axis control" class="Slide (strict)"("Value"=w372) -> ()  [unwired: 2 in, 2 out]
        n239 = property on="Theta-angle control" class="Slide (strict)"("Value"=w363) -> ()  [unwired: 2 in, 2 out]
      }
      frame #2 {
        # "This controller shall read the control from the mote and pass\nit to the crane"
        n240 = local read "u1"() -> (w380:sgl)
        n241 = local read "u2"() -> (w378:sgl)
        n242 = call "Saturation.vi"("Limit"=1.0, "Input"=0.0) -> ("Output"=w383:dbl)
        n243 = call "Saturation.vi"("Limit"=1.0, "Input"=w380) -> ("Output"=w385:dbl)
        n244 = call "Saturation.vi"("Limit"=1.0, "Input"=w378) -> ("Output"=w381:dbl)
        n245 = property on="Theta-angle control" class="Slide (strict)"("Value"=w381) -> ()  [unwired: 2 in, 2 out]
        n246 = property on="Z-axis control" class="Slide (strict)"("Value"=w383) -> ()  [unwired: 2 in, 2 out]
        n247 = property on="X-axis control" class="Slide (strict)"("Value"=w385) -> ()  [unwired: 2 in, 2 out]
      }
    }
    "Controller Description" <- w137
    n248 = node-c288() -> ()  [unwired: 1 in, 1 out]
    "X - Motor On/Off" <- "X-Motor On/Off"
    "Numeric" <- "X-axis control"
    "Theta - Motor On/Off" <- "T-Motor On/Off"
    "Numeric 2" <- "Theta-angle control"
    "Z - Motor On/Off" <- "Z-Motor On/Off"
    "Numeric 3" <- "Z-axis control"
  }
  n249 = call "CloseSF.vi"("error out"=w13, "connection ID"=w14) -> ()  [unwired: 1 in]
  n250 = node-c288(w19) -> ()  [unwired: 1 out]
